vi "Create directory.vi"(8 "error in (no error)":errorcluster, 10 "Directory":string, 11 "FTP in":refnum<class "FTP.lvclass">) -> (0 "error out":errorcluster, 3 "FTP out":refnum<class "FTP.lvclass">)   [LabVIEW 2016, in "RT Management.lvlib" / "FTP.lvclass"]
uses:
  FTP.lvclass
  C:/GitHub/SystemManagementAndInformation/source/classes/File Transfer Behavior/File Transfer Behavior.lvclass
  FTP.lvclass/FTP.ctl
  Get Session.vi
  <vilib>/Utility/error.llb/Trim Whitespace.vi
  File Transfer Behavior/File Transfer Behavior.lvclass
  <vilib>/FTP/NI_FTP.lvlib
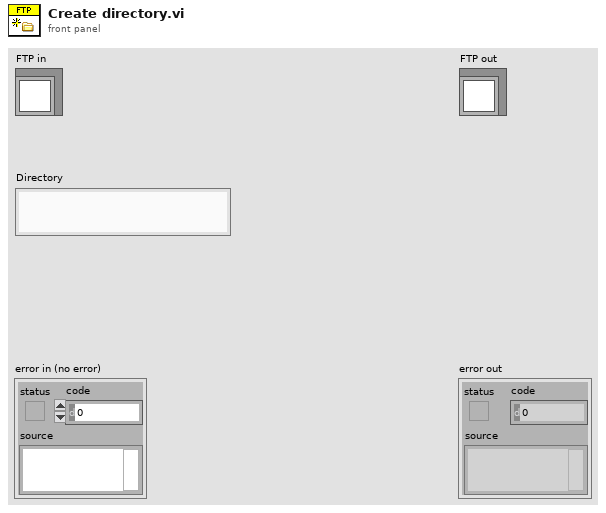
[diagram p1: front panel]
types:
  T1 = typedef "NI_FTP.lvlib/FTP Session.ctl" = refnum<k5>
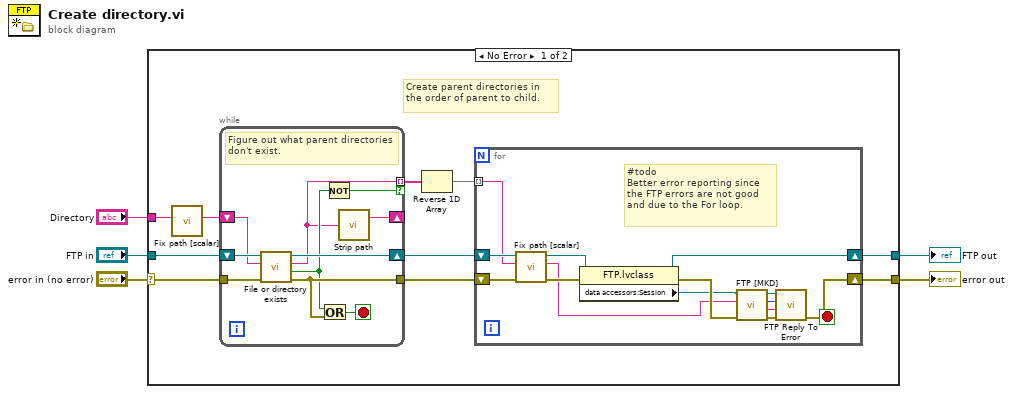
[diagram p0: block diagram]
diagram:
  n1 = case shown="No Error" "error in (no error)" {
    selector: "error in (no error)" -> [w9 w41]
    tunnel: "FTP in" -> [w13 w40]
    tunnel: "Directory" -> [w7 _]
    tunnel: [w8 w41] -> w1
    tunnel: [w10 w40] -> w2
    frame No Error {
      # "Create parent directories in the order of parent to child."
      n2 = call "Fix path [scalar].vi"("Path in"=w7) -> ("Path out"=w6:string)  [unwired: 8 in, 2 out]
      n3 = while {
        tunnel: [w35] -> w14
        tunnel: w9 -> [w38]
        tunnel: [w32] -> w12 mode=indexing if=w30
        shift-right: [w31] -> _
        shift-left: w6 -> [w36]
        shift-right: [w39] -> w15
        shift-left: w13 -> [w37]
        stop <- w34 stop-if-true
        # "Figure out what parent directories don't exist."
        n4 = call-dynamic "File or directory exists.vi"("error in (no error)"=w38, "Path"=w36, "FTP in"=w37) -> ("error out"=w35:errorcluster, "Exists?"=w33:bool, "Path out (dup)"=w32:string, "FTP out"=w39:refnum<class "FTP.lvclass">)  [unwired: 4 in, 1 out]
        n5 = Or(x=w33, y=w35) -> (x .or. y?=w34:bool)
        n6 = Not(x=w33) -> (.not. x?=w30:bool)
        n7 = call "Strip path.vi"("Path"=w32) -> ("Stripped path"=w31:string)  [unwired: 2 in, 1 out]
      }
      n8 = Reverse 1D Array(array=w12) -> (reversed array=w11:string[])
      n9 = for {
        tunnel: w11 -> [w27] mode=indexing
        shift-right: [w24] -> w10
        shift-left: w15 -> [w29]
        shift-right: [w17] -> w8
        shift-left: w14 -> [w28]
        stop <- w17 stop-if-true
        # "#todo\nBetter error reporting since the FTP errors are not good and due to the For loop."
        n10 = call "Fix path [scalar].vi"("error in (no error)"=w28, "Path in"=w27, "File Transfer Behavior in"=w29) -> ("error out"=w26:errorcluster, "Path out"=w18:string, "File Transfer Behavior out"=w25:refnum<class "FTP.lvclass">)  [unwired: 6 in]
        n11 = property class="FTP.lvclass"(reference=w25, error in=w26) -> (reference out=w24:refnum<class "FTP.lvclass">, error out=w20:errorcluster, "data accessors:Session"=w19:T1)
        n12 = call <vilib>:"FTP [MKD].vi"("error in (no error)"=w20, "directory path"=w18, "ftp session"=w19) -> ("error out"=w16:errorcluster, "reply string"=w21:string, "reply code"=w22:i32, "ftp session out"=w23:T1)  [unwired: 5 in]
        n13 = call <vilib>:"FTP Reply To Error.vi"("error in (no error)"=w16, "reply string in"=w21, "reply code in"=w22, "ftp session"=w23) -> ("error out"=w17:errorcluster)  [unwired: 3 out]
      }
    }
    frame Error {
    }
  }
  "error out" <- w1
  "FTP out" <- w2
